vi "Material-PassFail-LineN.vi"(8 "error in (no error)":errorcluster, 10 "Line?":i32, 11 "Material-RunTest in":refnum<class "Material-RunTest.lvclass">) -> (0 "error out":errorcluster, 3 "Material-RunTest out":refnum<class "Material-RunTest.lvclass">)   [LabVIEW 2014, in "Material-RunTest.lvclass"]
uses:
  Material-RunTest.lvclass
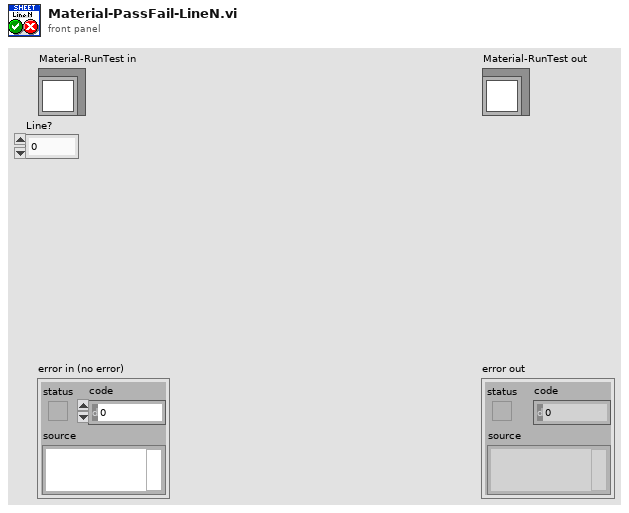
[diagram p1: front panel]
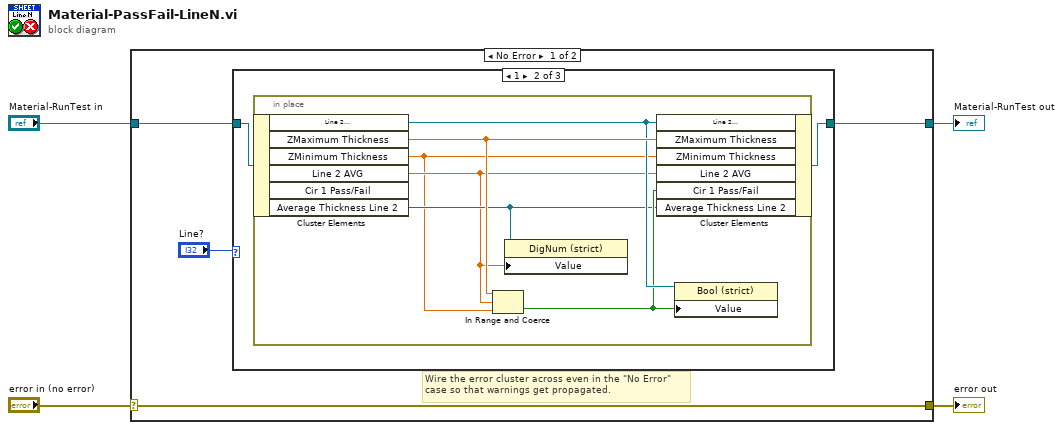
[diagram p0: block diagram]
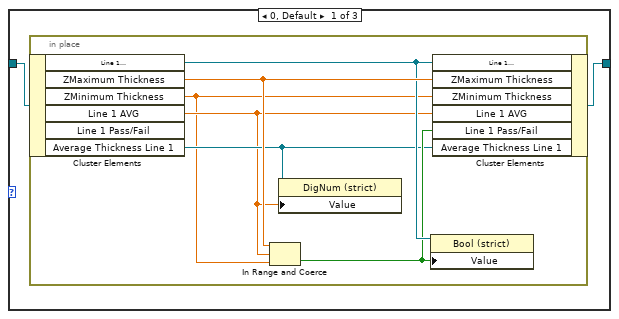
[diagram p2: hidden frame]
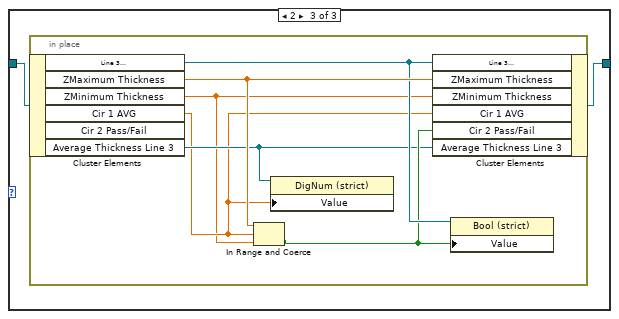
[diagram p3: hidden frame]
diagram:
  n1 = case shown="No Error" "error in (no error)" {
    selector: "error in (no error)" -> [w8 w34]
    tunnel: [w8 w34] -> w3
    tunnel: [w5 w33] -> w1
    tunnel: "Material-RunTest in" -> [w7 w33]
    frame No Error {
      # "Wire the error cluster across even in the \"No Error\"\ncase so that warnings get propagated."
      n2 = case shown="1" "Line?" {
        tunnel: w7 -> [w10 w18 w26]
        tunnel: [w9 w17 w25] -> w5
        frame 0, Default {
          n3 = in-place {
            n4 = in-place-cluster #1(w10) -> ("Line 1\ntest passed?"=w15:refnum<vi>, "ZMaximum Thickness"=w16:dbl, "ZMinimum Thickness"=w11:dbl, "Line 1 AVG"=w12:dbl, "Average Thickness Line 1"=w13:refnum<vi>)  [unwired: 1 out]
            n5 = In Range and Coerce(upper limit=w16, x=w12, lower limit=w11) -> (In Range?=w14:bool)  [unwired: 1 out]
            n6 = property class="DigNum (strict)"(reference=w13, "Value"=w12) -> ()  [unwired: 1 in, 2 out]
            n7 = property class="Bool (strict)"(reference=w15, "Value"=w14) -> ()  [unwired: 1 in, 2 out]
            n8 = in-place-cluster #1("Line 1\ntest passed?"=w15, "ZMaximum Thickness"=w16, "ZMinimum Thickness"=w11, "Line 1 AVG"=w12, "Line 1 Pass/Fail"=w14, "Average Thickness Line 1"=w13) -> (w9:refnum<class "Material-RunTest.lvclass">)
          }
        }
        frame 1 {
          n9 = in-place {
            n10 = in-place-cluster #2(w18) -> ("Line 2\ntest passed?"=w23:refnum<vi>, "ZMaximum Thickness"=w24:dbl, "ZMinimum Thickness"=w19:dbl, "Line 2 AVG"=w20:dbl, "Average Thickness Line 2"=w21:refnum<vi>)  [unwired: 1 out]
            n11 = In Range and Coerce(upper limit=w24, x=w20, lower limit=w19) -> (In Range?=w22:bool)  [unwired: 1 out]
            n12 = property class="DigNum (strict)"(reference=w21, "Value"=w20) -> ()  [unwired: 1 in, 2 out]
            n13 = in-place-cluster #2("Line 2\ntest passed?"=w23, "ZMaximum Thickness"=w24, "ZMinimum Thickness"=w19, "Line 2 AVG"=w20, "Cir 1 Pass/Fail"=w22, "Average Thickness Line 2"=w21) -> (w17:refnum<class "Material-RunTest.lvclass">)
            n14 = property class="Bool (strict)"(reference=w23, "Value"=w22) -> ()  [unwired: 1 in, 2 out]
          }
        }
        frame 2 {
          n15 = in-place {
            n16 = in-place-cluster #3(w26) -> ("Line 3\ntest passed?"=w31:refnum<vi>, "ZMaximum Thickness"=w32:dbl, "ZMinimum Thickness"=w27:dbl, "Cir 1 AVG"=w28:dbl, "Average Thickness Line 3"=w29:refnum<vi>)  [unwired: 1 out]
            n17 = In Range and Coerce(upper limit=w32, x=w28, lower limit=w27) -> (In Range?=w30:bool)  [unwired: 1 out]
            n18 = property class="DigNum (strict)"(reference=w29, "Value"=w28) -> ()  [unwired: 1 in, 2 out]
            n19 = in-place-cluster #3("Line 3\ntest passed?"=w31, "ZMaximum Thickness"=w32, "ZMinimum Thickness"=w27, "Cir 1 AVG"=w28, "Cir 2 Pass/Fail"=w30, "Average Thickness Line 3"=w29) -> (w25:refnum<class "Material-RunTest.lvclass">)
            n20 = property class="Bool (strict)"(reference=w31, "Value"=w30) -> ()  [unwired: 1 in, 2 out]
          }
        }
      }
    }
    frame Error {
    }
  }
  "error out" <- w3
  "Material-RunTest out" <- w1
